vi "GettingData(Temp&Viscosity).vi"() -> ()   [LabVIEW 2020]
uses:
  <vilib>/Instr/_visa.llb/VISA Open Access Mode.ctl
panel:
  out "length":i32
  out "element":string
  out "Viscosity":dbl
  out "Temperature":dbl
  in  "stop":bool
  in  "VISA resource name":refnum<visa-resource-name>
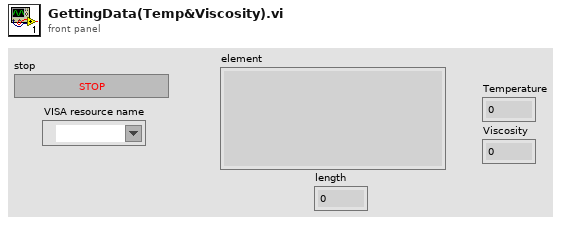
[diagram p1: front panel]
types:
  T1 = typedef "VISA Open Access Mode.ctl" = u32
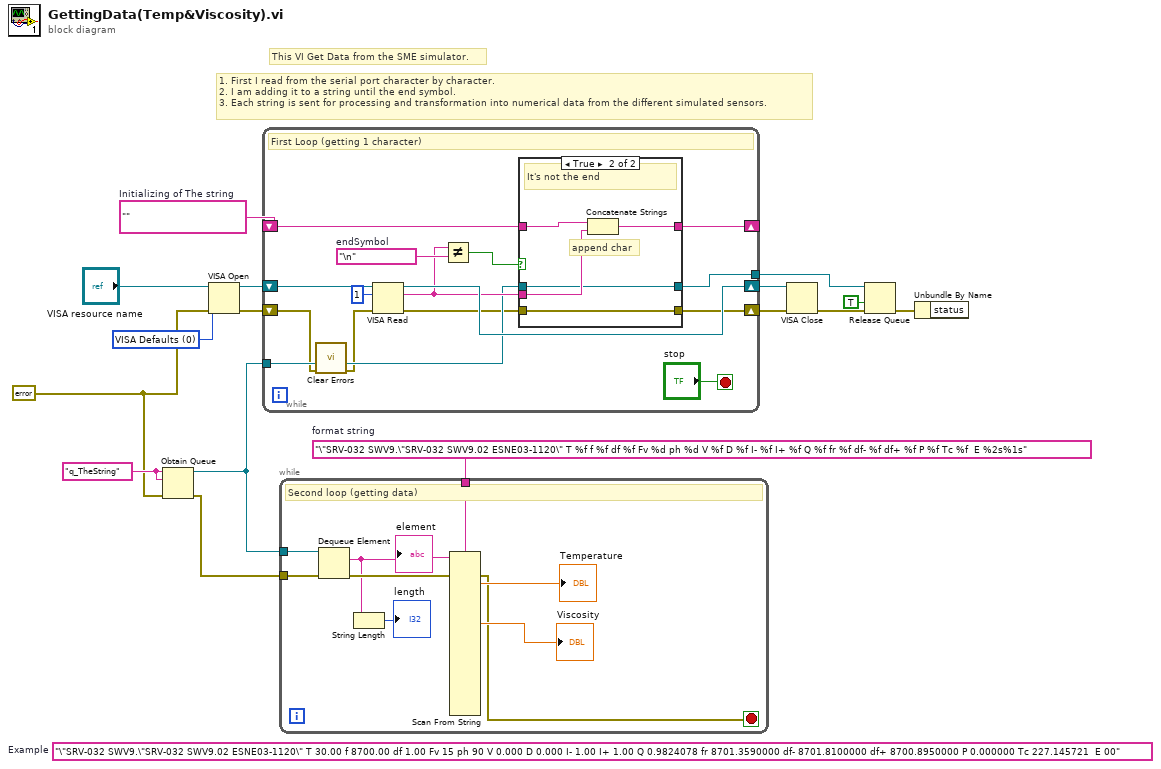
[diagram p0: block diagram]
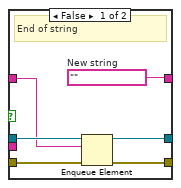
[diagram p2: hidden frame]
diagram:
  w1 = T1 0 items=["VISA Defaults"=0, "Exclusive Lock"=1, "Load Configured Settings"=4] ("Access Mode")
  w4 = ""  # Initializing of The string
  w6 = errorcluster {"status"=FALSE, "code"=0, "source"=""} ("error in (no error)")
  w7 = "\"SRV-032 SWV9.\"SRV-032 SWV9.02 ESNE03-1120\" T %f f %f df %f Fv %d ph %d V %f D %f I- %f I+ %f Q %f fr %f df- %f df+ %f P %f Tc %f  E %2s%1s"  # format string
  (unwired) "\"SRV-032 SWV9.\"SRV-032 SWV9.02 ESNE03-1120\" T 30.00 f 8700.00 df 1.00 Fv 15 ph 90 V 0.000 D 0.000 I- 1.00 I+ 1.00 Q 0.9824078 fr 8701.3590000 df- 8701.8100000 df+ 8700.8950000 P 0.000000 Tc 227.145721  E 00"  # Example
  w11 = "q_TheString" ("name (unnamed)")
  # "1. First I read from the serial port character by character.\n2. I am adding it to a string until the end symbol.\n3. Each string is sent for processing and transformation into numerical data from the different simulated sensors."
  # "This VI Get Data from the SME simulator."
  n1 = Obtain Queue(name (unnamed)=w11, element data type=w11, error in (no error)=w6) -> (queue out=w10:refnum<queue>, error out=w5:errorcluster)  [unwired: 2 in, 1 out]
  n2 = VISA Open(access mode=w1, error in (no error)=w6, VISA resource name="VISA resource name") -> (VISA resource name=w13:refnum<visa-resource-name>, error out=w12:errorcluster)  [unwired: 2 in]
  n3 = while {
    shift-right: [w31] -> w16
    shift-left: w13 -> [w30]
    shift-right: [w20] -> w15
    shift-left: w12 -> [w18]
    shift-right: [w23] -> _
    shift-left: w4 -> [w27]
    tunnel: w10 -> [w22]
    tunnel: [w19] -> w8
    stop <- "stop" stop-if-true
    w26 = "\n"  # endSymbol
    # "First Loop (getting 1 character)"
    n4 = call <vilib>:"Clear Errors.vi"("error in (no error)"=w18) -> ("error out"=w17:errorcluster)  [unwired: 5 in, 1 out]
    n5 = VISA Read(VISA resource name=w30, byte count=u32 1, error in (no error)=w17) -> (VISA resource name out=w31:refnum<visa-resource-name>, read buffer=w25:string, error out=w21:errorcluster)  [unwired: 1 out]
    n6 = Not Equal?(x=w25, y=w26) -> (x != y?=w24:bool)
    n7 = case shown="True" w24 {
      tunnel: w27 -> [w33 w42]
      tunnel: w25 -> [_ w41]
      tunnel: [w32 w40] -> w23
      tunnel: w22 -> [w37 w38]
      tunnel: w21 -> [w36 w39]
      tunnel: [w35 w39] -> w20
      tunnel: [w34 w38] -> w19
      frame False {
        w32 = ""  # New string
        # "End of string"
        n8 = Enqueue Element(queue=w37, element=w33, error in (no error)=w36) -> (queue out=w34:refnum<queue>, error out=w35:errorcluster)  [unwired: 1 in, 1 out]
      }
      frame True {
        # "append char"
        # "It's not the end"
        n9 = Concatenate Strings(w42, w41) -> (w40:string)
      }
    }
  }
  n10 = while {
    tunnel: w10 -> [w51]
    tunnel: w7 -> [w50]
    tunnel: w5 -> [w47]
    stop <- w45 stop-if-true
    # "Second loop (getting data)"
    n11 = Dequeue Element(queue=w51, error in (no error)=w47) -> (element=w44:string, error out=w46:errorcluster)  [unwired: 1 in, 2 out]
    "element" <- w44
    n12 = String Length(string=w44) -> (length=→"length":i32)
    n13 = Scan From String(format string=w50, input string=w44, error in=w46) -> (error out=w45:errorcluster, output 1=→"Temperature":dbl, output 6=→"Viscosity":dbl)  [unwired: 33 in, 2 out]
  }
  n14 = VISA Close(VISA resource name=w16, error in (no error)=w15) -> (error out=w9:errorcluster)
  n15 = Release Queue(queue=w8, force destroy? (F)=TRUE, error in (no error)=w9) -> (error out=w2:errorcluster)  [unwired: 2 out]
  n16 = Unbundle By Name(w2) -> ()  [unwired: 1 out]
